vi "Digitial Integrator Set Gain.vi"(8 "error in (no error)":errorcluster, 10 "Gain":i16(slide)=1 min=0 max=9 step=1 scale=0.0..9.0, 11 "VISA resource name":refnum<visa-resource-name>) -> (0 "error out":errorcluster, 3 "VISA resource name dup":refnum<visa-resource-name>)   [LabVIEW 2021]
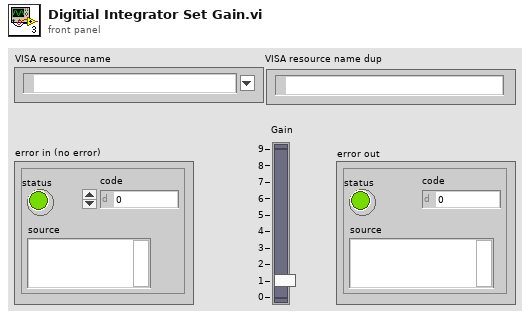
[diagram p1: front panel]
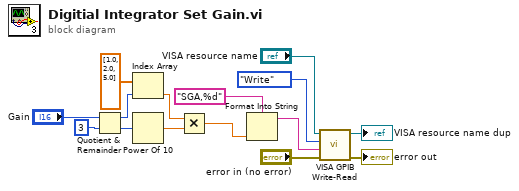
[diagram p0: block diagram]
diagram:
  n1 = Quotient & Remainder(x="Gain", y=i16 3) -> (x-y*floor(x/y)=w9:i16, floor(x/y)=w7:i16)
  n2 = Index Array(array=dbl[] [1.0, 2.0, 5.0], index=w9) -> (element=w5:dbl)
  n3 = Power Of 10(x=w7) -> (10^x=w6:dbl)
  n4 = Multiply(x=w5, y=w6) -> (x*y=w4:dbl)
  n5 = Format Into String(format string="SGA,%d", w4) -> (resulting string=w2:string)  [unwired: 2 in, 1 out]
  n6 = call "VISA GPIB Write-Read.vi"("error in (no error)"="error in (no error)", "Command"=w2, "Action"=enum16{"Write", "Read", "Write & Read"}."Write", "VISA resource name"="VISA resource name") -> ("error out"=→"error out":errorcluster, "dup VISA Session"=→"VISA resource name dup":refnum<visa-resource-name>)  [unwired: 4 in, 2 out]
